vi "Update_Selected_Space_File.vi"(1 "Selected Space File Name":string, 2 "Traverse Setup":string) -> ()   [LabVIEW 2013]
uses:
  Globals/Constants_global.vi
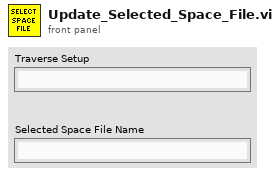
[diagram p1: front panel]
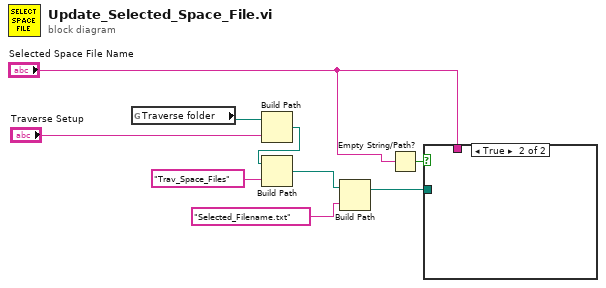
[diagram p0: block diagram]
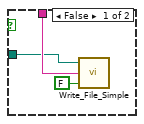
[diagram p2: hidden frame]
diagram:
  n1 = global read "Constants_global.vi" "Traverse folder"() -> (w7:path)
  n2 = Build Path(base path=w7, name or relative path="Traverse Setup") -> (appended path=w4:path)
  n3 = Build Path(base path=w4, name or relative path="Trav_Space_Files" ("Substring")) -> (appended path=w5:path)
  n4 = Build Path(base path=w5, name or relative path="Selected_Filename.txt" ("Substring")) -> (appended path=w9:path)
  n5 = Empty String/Path?(string/path="Selected Space File Name") -> (empty?=w2:bool)
  n6 = case shown="True" w2 {
    tunnel: "Selected Space File Name" -> [w11 _]
    tunnel: w9 -> [w10 _]
    frame False {
      n7 = call "Write_File_Simple.vi"("append to file? (new file:F)"=FALSE, "character string"=w11, "file path"=w10) -> ()  [unwired: 2 out]
    }
    frame True {
    }
  }
